vi "WPI_RobotDriveMotors_3005_Fuel.vi"(8 "error in":errorcluster, 9 "RightSpeed":dbl, 10 "LeftSpeed":dbl, 11 "RobotDriveDevRef":T1={"DevStatus"={"status"=FALSE, "code"=0, "source"=""}, "Motors[]"=[], "Square Inputs"=FALSE, "Max Output"=1.0}) -> (0 "error out":errorcluster, 2 "Motor Values":dbl[](array[numeric]), 3 "RobotDriveDevRef":T1={"DevStatus"={"status"=FALSE, "code"=0, "source"=""}, "Motors[]"=[], "Square Inputs"=FALSE, "Max Output"=1.0})   [LabVIEW 2016]
doc: "Determines the motor configuration and sends the speed values to the appropriate motors.\n\nThis software is licensed. Open the labview\\readme\\WPI Robotics Library Open Source License.txt file for more information."
uses:
  <vilib>/Rock Robotics/WPI/RobotDrive/WPI_RobotDriveDevRef.ctl
  <vilib>/Rock Robotics/WPI/MotorControl/WPI_MotorControlDeviceRef.ctl
  <vilib>/Rock Robotics/WPI/MotorControl/WPI_MotorControlType.ctl
  <vilib>/Rock Robotics/SystemInterfaces/DIO/FPGA_DIOPWMChannel.ctl
  <vilib>/Rock Robotics/WPI/PWM/WPI_PWMDeadband.ctl
  <vilib>/Rock Robotics/WPI/RobotDrive/WPI_RobotDriveSafetyCheck.vi
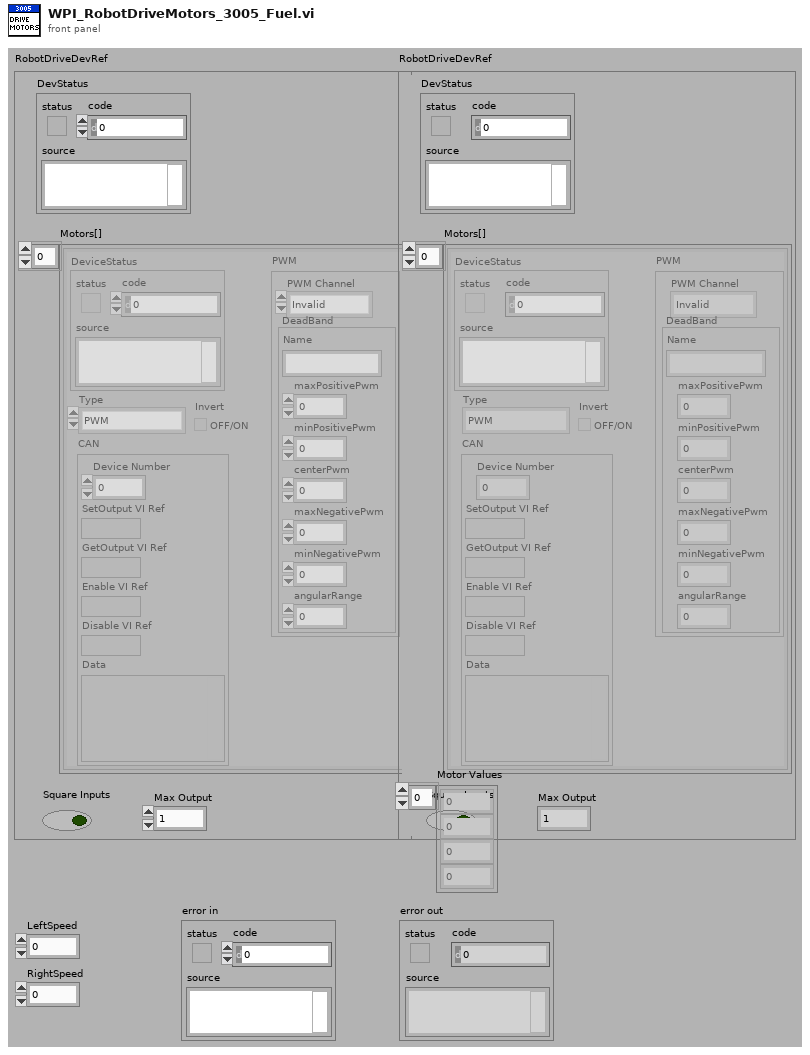
[diagram p1: front panel]
types:
  T1 = typedef "WPI_RobotDriveDevRef.ctl" = cluster{"DevStatus":errorcluster, "Motors[]":T2[], "Square Inputs":bool, "Max Output":dbl}
  T2 = typedef "WPI_MotorControlDeviceRef.ctl" = cluster{"DeviceStatus":errorcluster, "Type":T3, "PWM":cluster{"PWM Channel":T4, "DeadBand":T5}, "CAN":cluster{"Device Number":u8, "SetOutput VI Ref":variant, "GetOutput VI Ref":variant, "Enable VI Ref":variant, "Disable VI Ref":variant, "Data":variant}, "Invert":bool}
  T3 = typedef "WPI_MotorControlType.ctl" = enum16{"PWM", "CAN"}
  T4 = typedef "FPGA_DIOPWMChannel.ctl" = enum8{"PWM 0", "PWM 1", "PWM 2", "PWM 3", "PWM 4", "PWM 5", "PWM 6", "PWM 7", "PWM 8", "PWM 9", "PWM MXP 0", "PWM MXP 1", "PWM MXP 2", "PWM MXP 3", "PWM MXP 4", "PWM MXP 5", "PWM MXP 6", "PWM MXP 7", "PWM MXP 8", "PWM MXP 9", "Invalid"}
  T5 = typedef "WPI_PWMDeadband.ctl" = cluster{"Name":string, "maxPositivePwm":i32, "minPositivePwm":i32, "centerPwm":i32, "maxNegativePwm":i32, "minNegativePwm":i32, "angularRange":u16}
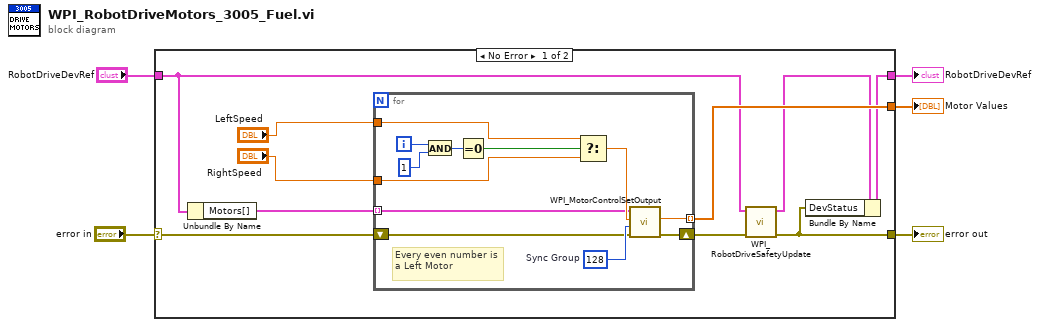
[diagram p0: block diagram]
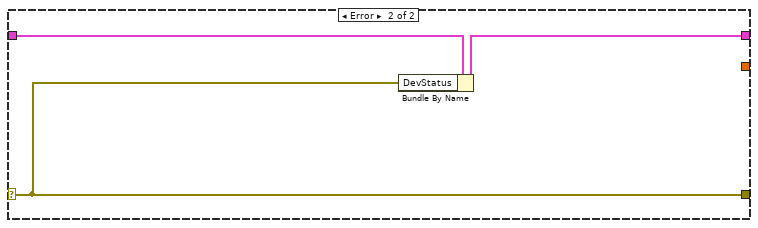
[diagram p2: hidden frame]
diagram:
  n1 = case shown="No Error" "error in" {
    selector: "error in" -> [w8 w28]
    tunnel: [w13 _] -> w5
    tunnel: "RobotDriveDevRef" -> [w12 w30]
    tunnel: [w10 w29] -> w3
    tunnel: [w9 w28] -> w2
    frame No Error {
      n2 = Unbundle By Name(w12) -> ("Motors[]"=w15:T2[])
      n3 = for {
        tunnel: [w27] -> w13 mode=indexing
        tunnel: w15 -> [w21] mode=indexing
        shift-right: [w19] -> w14
        shift-left: w8 -> [w18]
        tunnel: "LeftSpeed" -> [w17]
        tunnel: "RightSpeed" -> [w16]
        i -> [w26]
        w20 = u8 128  # Sync Group
        # "Every even number is a Left Motor"
        n4 = And(x=w26, y=1) -> (x .and. y?=w24:i32)
        n5 = Equal To 0?(x=w24) -> (x = 0?=w23:bool)
        n6 = Select(t=w17, s=w23, f=w16) -> (s? t:f=w22:dbl)
        n7 = call <vilib>:"WPI_MotorControlSetOutput.vi"("error in (no error)"=w18, "options"=w20, "Output"=w22, "MotorControlDevRef"=w21) -> ("error out"=w19:errorcluster, "Motor Output"=w27:dbl)  [unwired: 6 out]
      }
      n8 = call <vilib>:"WPI_RobotDriveSafetyUpdate.vi"("error in (no error)"=w14, "RobotDriveDevRef"=w12) -> ("error out"=w9:errorcluster, "RobotDriveDevRef"=w11:T1)  [unwired: 8 out]
      n9 = Bundle By Name(cluster=w11, "DevStatus"=w9) -> (w10:T1)
    }
    frame Error {
      n10 = Bundle By Name(cluster=w30, "DevStatus"=w28) -> (w29:T1)
    }
  }
  "RobotDriveDevRef" <- w3
  "error out" <- w2
  "Motor Values" <- w5
